vi "app append to log.vi"(11 "log line to append":string) -> ()   [LabVIEW 2013]
uses:
  app global state actions.ctl
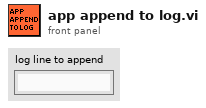
[diagram p1: front panel]
types:
  T1 = typedef "app global state actions.ctl" = enum16{"get cluster", "set cluster", "set current sweep", "set field value", "set ramping", "set sweeping", "append log", "clear log", "set finished"}
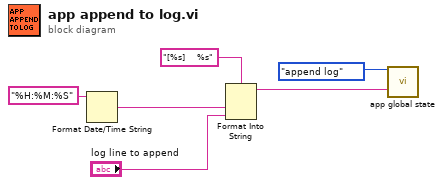
[diagram p0: block diagram]
diagram:
  n1 = Format Date/Time String(time format string (%c)="%H:%M:%S") -> (date/time string=w4:string)  [unwired: 2 in]
  n2 = Format Into String(format string="[%s]    %s", w4, "log line to append") -> (resulting string=w2:string)  [unwired: 2 in, 1 out]
  n3 = call "app global state.vi"("action"=app_global_state_actions."append log" ("app global state actions"), "log line to append"=w2) -> ()  [unwired: 17 in, 1 out]
